vi "U8arrayToMeasurement.vi"(4 "payload":u8[](array[numeric]), 5 "factor 4":dbl=1.0 format="%#_13g", 6 "factor 3":dbl=1.0 format="%#_13g", 7 "factor 2":dbl=1.0 format="%#_13g", 8 "factor 1":dbl=1.0 format="%#_13g") -> (0 "Meas 4":dbl, 1 "Meas 3":dbl, 2 "Meas 1":dbl, 3 "Meas 2":dbl)   [LabVIEW 2021]
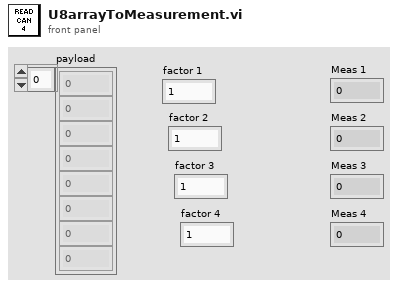
[diagram p1: front panel]
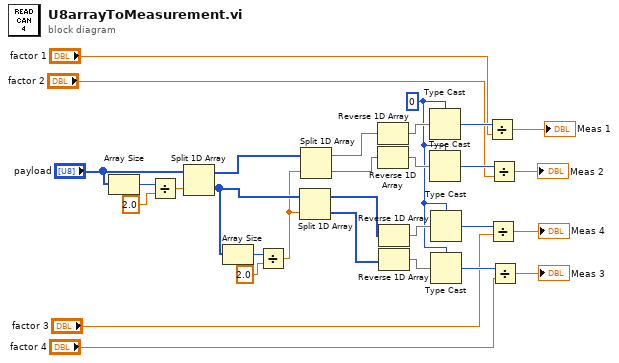
[diagram p0: block diagram]
diagram:
  w1 = u16 0
  n1 = Array Size(array="payload") -> (size(s)=w25:i32)
  n2 = Divide(x=w25, y=2.0) -> (x/y=w27:dbl)
  n3 = Split 1D Array(array="payload", index=w27) -> (first subarray=w18:u8[], second subarray=w16:u8[])
  n4 = Array Size(array=w16) -> (size(s)=w3:i32)
  n5 = Divide(x=w3, y=2.0) -> (x/y=w15:dbl)
  n6 = Split 1D Array(array=w16, index=w15) -> (first subarray=w7:u8[], second subarray=w6:u8[])
  n7 = Split 1D Array(array=w18, index=w15) -> (first subarray=w14:u8[], second subarray=w2:u8[])
  n8 = Reverse 1D Array(array=w14) -> (reversed array=w28:u8[])
  n9 = Reverse 1D Array(array=w2) -> (reversed array=w29:u8[])
  n10 = Reverse 1D Array(array=w7) -> (reversed array=w11:u8[])
  n11 = Reverse 1D Array(array=w6) -> (reversed array=w12:u8[])
  n12 = Type Cast(type=w1, x=w28) -> (*(type *) &x=w30:u16)
  n13 = Type Cast(type=w1, x=w29) -> (*(type *) &x=w23:u16)
  n14 = Type Cast(type=w1, x=w11) -> (*(type *) &x=w13:u16)
  n15 = Type Cast(type=w1, x=w12) -> (*(type *) &x=w10:u16)
  n16 = Divide(x=w30, y="factor 1") -> (x/y=→"Meas 1":dbl)
  n17 = Divide(x=w13, y="factor 3") -> (x/y=→"Meas 4":dbl)
  n18 = Divide(x=w23, y="factor 2") -> (x/y=→"Meas 2":dbl)
  n19 = Divide(x=w10, y="factor 4") -> (x/y=→"Meas 3":dbl)
